vi "Read Source.vi"(8 "Error In":errorcluster, 11 "Node In":refnum<class "Comment.lvclass">) -> (0 "Error Out":errorcluster, 2 "Source":string, 3 "Node Out":refnum<class "Comment.lvclass">)   [LabVIEW 2018, in "Toolkit.lvlib" / "Nodes.lvlib" / "Comment.lvclass"]
uses:
  Comment.lvclass
  Comment.lvclass/Comment.ctl
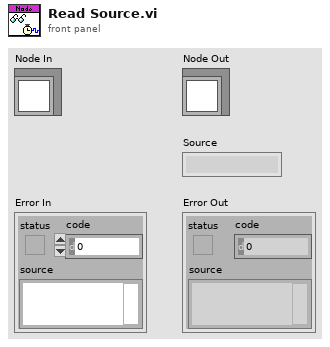
[diagram p1: front panel]
types:
  T1 = typedef "Toolkit.lvlib/Delimiters.ctl" = cluster{"Close":string, "Open":string}
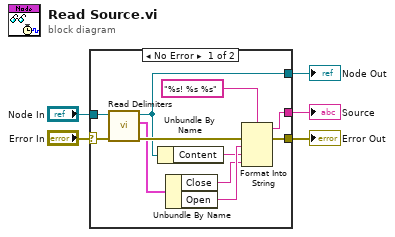
[diagram p0: block diagram]
diagram:
  n1 = case shown="No Error" "Error In" {
    selector: "Error In" -> [w16 w17]
    tunnel: "Node In" -> [w15 w18]
    tunnel: [w6 _] -> w3
    tunnel: [w11 w17] -> w2
    tunnel: [w13 w18] -> w1
    frame No Error {
      n2 = call-dynamic "Read Delimiters.vi"("Error In"=w16, "Node In"=w15) -> ("Error Out"=w14:errorcluster, "Delimiters"=w12:T1, "Node Out"=w13:refnum<class "Comment.lvclass">)  [unwired: 7 in]
      n3 = Unbundle By Name(w13) -> ("Content"=w8:string)
      n4 = Unbundle By Name(w12) -> ("Close"=w7:string, "Open"=w9:string)
      n5 = Format Into String(format string="%s! %s %s", error in=w14, w9, w8, w7) -> (resulting string=w6:string, error out=w11:errorcluster)  [unwired: 1 in]
    }
    frame Error {
    }
  }
  "Error Out" <- w2
  "Node Out" <- w1
  "Source" <- w3
